vi "Write GEI status.vi"(8 "error in (no error)":errorcluster, 10 "GEI status":T1={"OBJECT"="", "OBSERVER"="", "CTRLINTE"="GEI", "PROJID"="", "SYNCMODE"="ASYNC", "INSTMODE"="PHOT", "FILTER"="CLEAR", "OBSTYPE"="", "GUIVRSN"="V0.0.0", "COMMENT"="", "broker"="GEI", "timestamp"="0000-00-00T00:00:00.0", "CHANNEL 1"=TRUE, "CHANNEL 2"=FALSE, "CHANNEL 3"=FALSE, "CHANNEL 4"=FALSE, "TCSMODE"=TRUE}, 11 "S4GEI in":refnum<class "S4GEI.lvclass">) -> (0 "error out":errorcluster, 3 "S4GEI out":refnum<class "S4GEI.lvclass">)   [LabVIEW 2018, in "S4GEI.lvclass"]
uses:
  S4GEI.lvclass
  S4GEI.lvclass/S4GEI.ctl
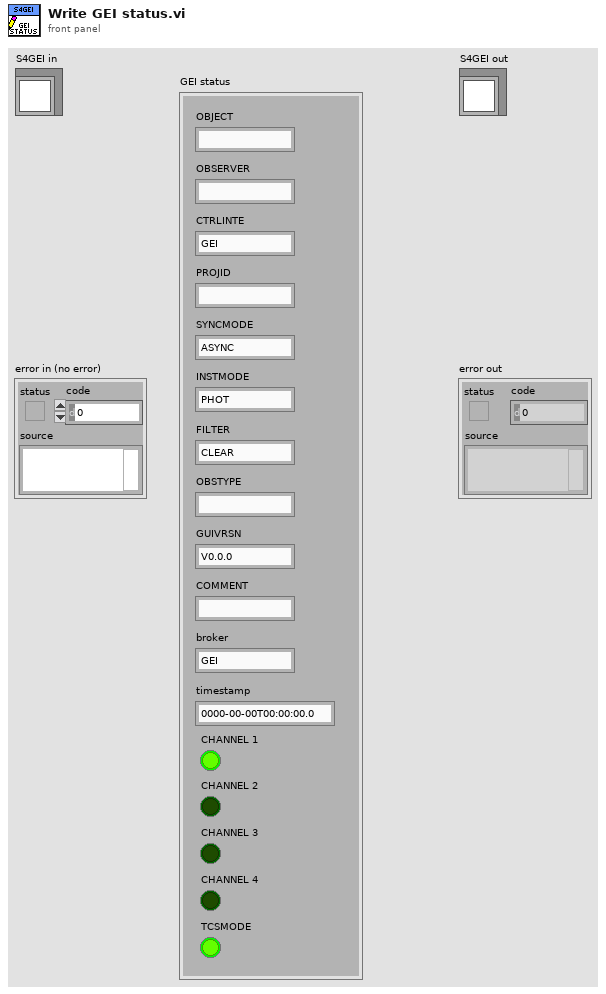
[diagram p1: front panel]
types:
  T1 = cluster{"OBJECT":string, "OBSERVER":string, "CTRLINTE":string, "PROJID":string, "SYNCMODE":string, "INSTMODE":string, "FILTER":string, "OBSTYPE":string, "GUIVRSN":string, "COMMENT":string, "broker":string, "timestamp":string, "CHANNEL 1":bool, "CHANNEL 2":bool, "CHANNEL 3":bool, "CHANNEL 4":bool, "TCSMODE":bool}
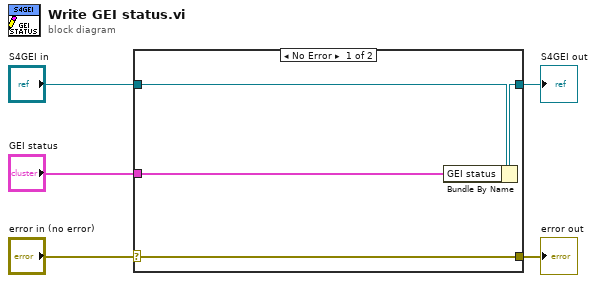
[diagram p0: block diagram]
diagram:
  n1 = case shown="No Error" "error in (no error)" {
    selector: "error in (no error)" -> [w9 w10]
    tunnel: [w9 w10] -> w4
    tunnel: [w7 w11] -> w2
    tunnel: "S4GEI in" -> [w8 w11]
    tunnel: "GEI status" -> [w6 _]
    frame No Error {
      n2 = Bundle By Name(cluster=w8, "GEI status"=w6) -> (w7:refnum<class "S4GEI.lvclass">)
    }
    frame Error {
    }
  }
  "error out" <- w4
  "S4GEI out" <- w2
